vi "Tokenize String.vi"(5 "String (\"\")":string, 11 "Error In":errorcluster caption="エラー入力") -> (6 "Result":string[](array[string]), 15 "Error Out":errorcluster caption="エラー出力")   [LabVIEW 2020, in "Yokogawa GX Series.lvlib"]
doc: "Adds quote to string and concatenate to initial string."
uses:
  <instrlib>/Yokogawa GX Series/Yokogawa GX Series.lvlib
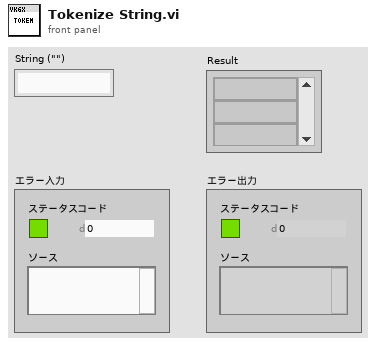
[diagram p1: front panel]
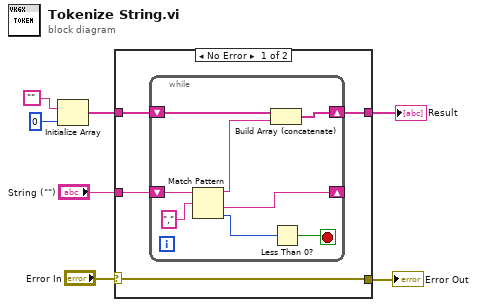
[diagram p0: block diagram]
diagram:
  n1 = Initialize Array("", 0) -> (w3:string[])
  n2 = case shown="No Error" "Error In" {
    selector: "Error In" -> [w9 w21]
    tunnel: [w9 w21] -> w7
    tunnel: w3 -> [w11 w20]
    tunnel: [w8 w20] -> w2
    tunnel: "String (\"\")" -> [w10 _]
    frame No Error {
      n3 = while {
        shift-right: [w17] -> w8
        shift-left: w11 -> [w18]
        shift-right: [w13] -> _
        shift-left: w10 -> [w16]
        stop <- w19 stop-if-true
        n4 = Match Pattern(string=w16, regular expression=",") -> (before substring=w14:string, after substring=w13:string, offset past match=w12:i32)  [unwired: 1 in, 1 out]
        n5 = Build Array (concatenate)(w18, w14) -> (w17:string[])
        n6 = Less Than 0?(x=w12) -> (x < 0?=w19:bool)
      }
    }
    frame Error {
    }
  }
  "Error Out" <- w7
  "Result" <- w2
